vi "Write Field Specs.vi"(8 "error in (no error)":errorcluster, 10 "Field Specs":T1[](array[typedef])=[{"Name"="Length", "Offset"=0, "Length"=1, "FieldType"=enum."Binary"}, {"Name"="MessageType", "Offset"=1, "Length"=1, "FieldType"=enum."Value"}, {"Name"="Time Offset", "Offset"=2, "Length"=4, "FieldType"=enum."Binary"}, {"Name"="Order Id", "Offset"=6, "Length"=8, "FieldType"=enum."Binary"}, {"Name"="Side Indicator", "Offset"=14, "Length"=1, "FieldType"=enum."Alphanumeric"}, {"Name"="Quantity", "Offset"=15, "Length"=4, "FieldType"=enum."Binary"}, {"Name"="Symbol", "Offset"=19, "Length"=6, "FieldType"=enum."PrintableAscii"}, {"Name"="Price", "Offset"=25, "Length"=8, "FieldType"=enum."BinaryLongPrice"}, {"Name"="Add Flags", "Offset"=33, "Length"=1, "FieldType"=enum."BitField"}], 11 "PitchMessage in":refnum<class "PitchMessage.lvclass">) -> (0 "error out":errorcluster, 3 "PitchMessage out":refnum<class "PitchMessage.lvclass">)   [LabVIEW 2022 SP3, in "PitchMessage.lvclass"]
uses:
  PitchMessage.lvclass
  FieldSpec.ctl
  PitchMessage.lvclass/PitchMessage.ctl
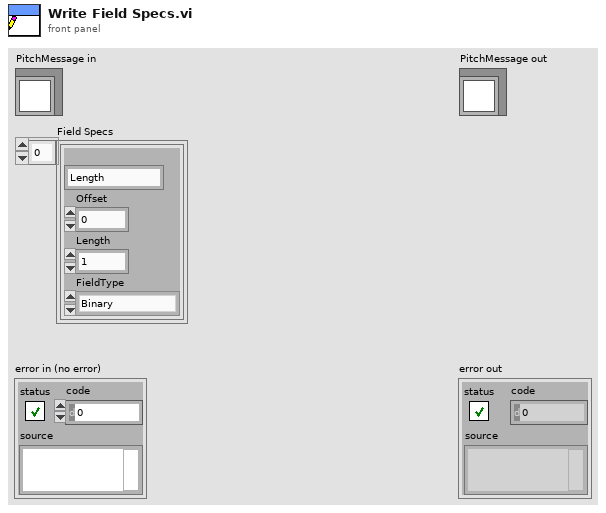
[diagram p1: front panel]
types:
  T1 = typedef "FieldSpec.ctl" = cluster{"Name":string, "Offset":i32, "Length":i32, "FieldType":enum16{"Alphanumeric", "Binary", "BinaryLongPrice", "BinaryShortPrice", "BitField", "PrintableAscii", "Value"}}
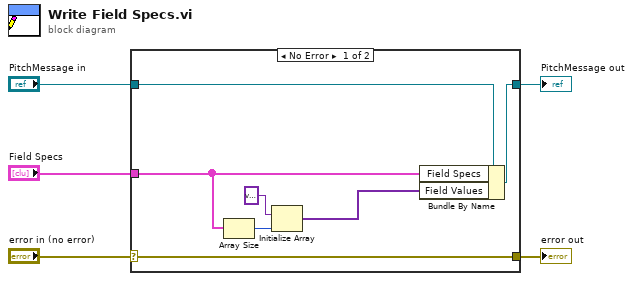
[diagram p0: block diagram]
diagram:
  n1 = case shown="No Error" "error in (no error)" {
    selector: "error in (no error)" -> [w12 w13]
    tunnel: [w12 w13] -> w4
    tunnel: [w10 w14] -> w2
    tunnel: "PitchMessage in" -> [w11 w14]
    tunnel: "Field Specs" -> [w7 _]
    frame No Error {
      n2 = Array Size(array=w7) -> (size(s)=w6:i32)
      n3 = Initialize Array(variant, w6) -> (w9:variant[])
      n4 = Bundle By Name(cluster=w11, "Field Specs"=w7, "Field Values"=w9) -> (w10:refnum<class "PitchMessage.lvclass">)
    }
    frame Error {
    }
  }
  "error out" <- w4
  "PitchMessage out" <- w2
